vi "Get Calibration Point Auto.vi"(0 "Manipulator Interface":T3, 1 "Diagonal factor":dbl min=0.0 max=1.0, 2 "Focus and Tracking":T1, 5 "error in":errorcluster, 7 "System of Reference Interface":T2, 12 "Dialog Indicator":refnum<vi>, 13 "Calibrate button":refnum<vi>) -> (14 "Distance [um]":dbl format="%.2f", 15 "Initial [pix]":cluster{"X":sgl, "Y":sgl}, 16 "Final [pix]":cluster{"X":sgl, "Y":sgl}, 17 "Initial Reference Point [um]":cluster{"X":dbl, "Y":dbl}, 18 "Final Reference Point [um]":cluster{"X":dbl, "Y":dbl}, 19 "error out":errorcluster)   [LabVIEW 2012, in "Targeting Unit.lvlib"]
uses:
  Targeting Unit.lvlib
  <vilib>/Analysis/Matrix/Datatypes/RealMatrix.ctl
  <vilib>/Analysis/Matrix/NI_Matrix.lvlib
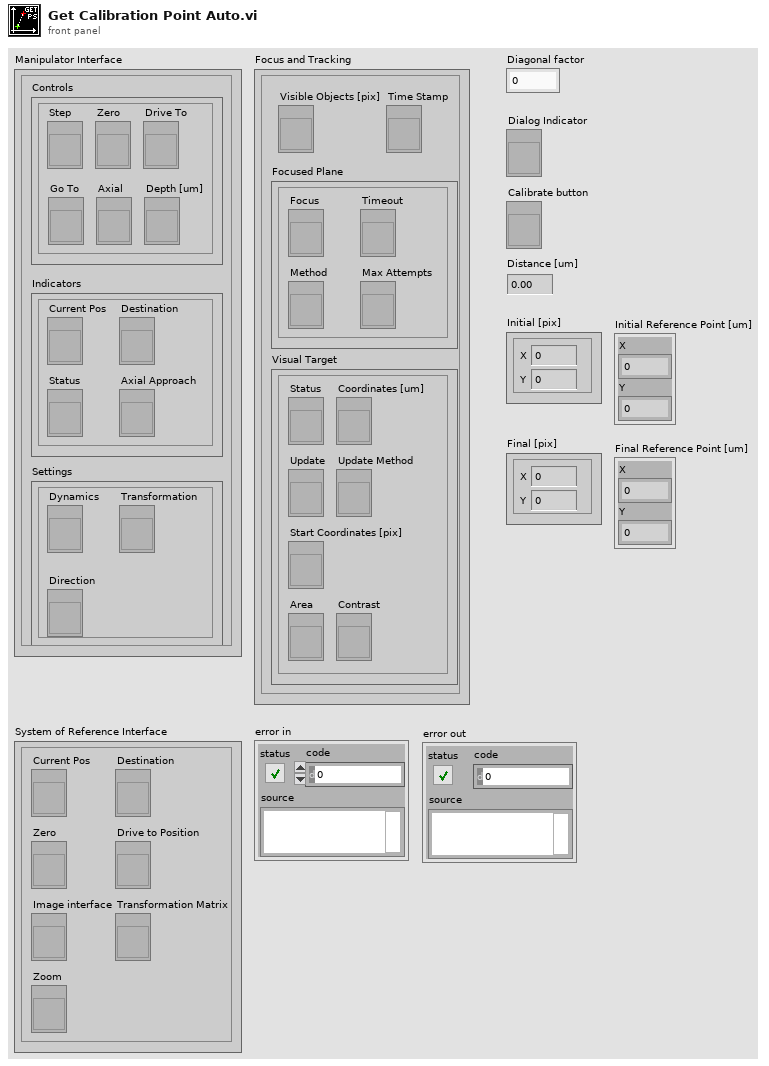
[diagram p1: front panel]
types:
  T1 = cluster{"Focused Plane":cluster{"Focus":refnum<vi>, "Timeout":refnum<vi>, "Max Attempts":refnum<vi>, "Method":refnum<vi>}, "Time Stamp":refnum<vi>, "Visual Target":cluster{"Coordinates [um]":refnum<vi>, "Status":refnum<vi>, "Update":refnum<vi>, "Update Method":refnum<vi>, "Start Coordinates [pix]":refnum<vi>, "Area":refnum<vi>, "Contrast":refnum<vi>}, "Visible Objects [pix]":refnum<vi>}
  T2 = cluster{"Current Pos":refnum<vi>, "Image interface":refnum<vi>, "Transformation Matrix":refnum<vi>, "Zero":refnum<vi>, "Destination":refnum<vi>, "Drive to Position":refnum<vi>, "Zoom":refnum<vi>}
  T3 = cluster{"Indicators":cluster{"Current Pos":refnum<vi>, "Destination":refnum<vi>, "Status":refnum<vi>, "Axial Approach":refnum<vi>}, "Settings":cluster{"Dynamics":refnum<vi>, "Transformation":refnum<vi>, "Direction":refnum<vi>}, "Controls":cluster{"Zero":refnum<vi>, "Step":refnum<vi>, "Drive To":refnum<vi>, "Go To":refnum<vi>, "Axial":refnum<vi>, "Depth [um]":refnum<vi>}}
  T4 = cluster{"X [um]":dbl, "Y [um]":dbl, "Z [um]":dbl}
  T5 = typedef "NI_Matrix.lvlib/RealMatrix.ctl" = dbl[][]
  T6 = cluster{"Area":dbl, "Centre of Mass":cluster{"X":dbl, "Y":dbl}, "Global Rectangle":cluster{"Left":dbl, "Top":dbl, "Right":dbl, "Bottom":dbl}, "Contrast":dbl}[]
  T7 = cluster{"Area":dbl, "Centre of Mass":cluster{"X":dbl, "Y":dbl}, "Global Rectangle":cluster{"Left":dbl, "Top":dbl, "Right":dbl, "Bottom":dbl}, "Contrast":dbl}
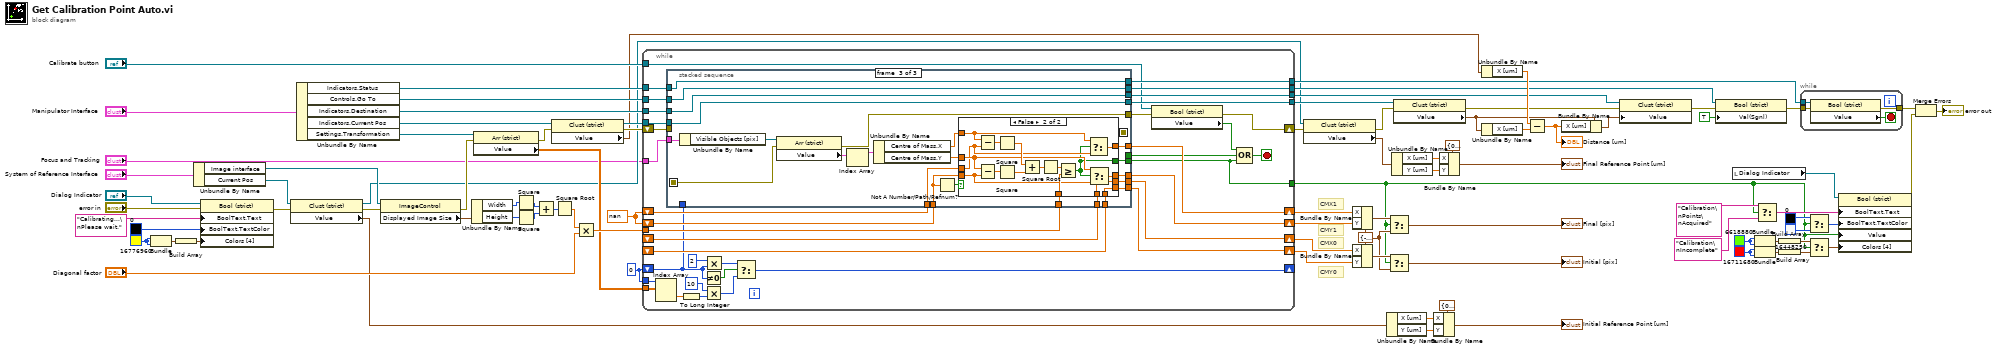
[diagram p0: block diagram]
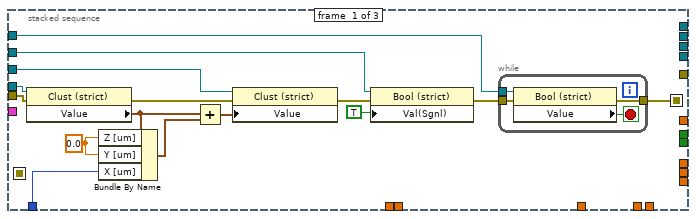
[diagram p2: hidden frame]
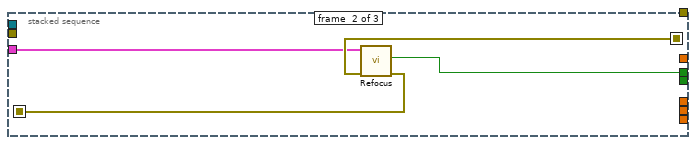
[diagram p3: hidden frame]
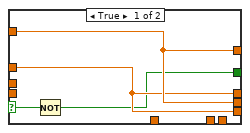
[diagram p4: hidden frame]
diagram:
  w31 = u32 16711680
  w28 = u32 6618880
  w41 = u32 16776960
  w13 = cluster{"X":i32, "Y":i32} {"X"=-1, "Y"=-1} ("Final [pix]")
  w86 = nan ("Numeric")
  w54 = 0 ("index (row)")
  # "CMY0"
  # "CMX0"
  # "CMY1"
  # "CMX1"
  n1 = Bundle(w41, w41) -> (w42:cluster{u32, u32})  [unwired: 1 in]
  n2 = Build Array(w42) -> (w38:cluster{u32, u32}[])
  n3 = Unbundle By Name("System of Reference Interface") -> ("Image interface"=w53:refnum<vi>, "Current Pos"=w46:refnum<vi>)
  n4 = property class="Bool (strict)"(reference="Dialog Indicator", error in="error in", "BoolText.Text"="Calibrating...\nPlease wait." ("Boolean Text.Text"), "BoolText.TextColor"=u32 0, "Colors [4]"=w38) -> (error out=w36:errorcluster)  [unwired: 1 out]
  n5 = property class="Clust (strict)"(reference=w46, error in=w36) -> (reference out=w43:refnum<vi>, error out=w47:errorcluster, "Value"=w11:T4)
  n6 = Unbundle By Name("Manipulator Interface") -> ("Indicators.Status"=w62:refnum<vi>, "Controls.Go To"=w63:refnum<vi>, "Indicators.Destination"=w67:refnum<vi>, "Indicators.Current Pos"=w76:refnum<vi>, "Settings.Transformation"=w74:refnum<vi>)
  n7 = property class="ImageControl"(reference=w53, error in=w47) -> (error out=w52:errorcluster, "Displayed Image Size"=w51:cluster{"Width":u32, "Height":u32})  [unwired: 1 out]
  n8 = Unbundle By Name(w51) -> ("Width"=w83:u32, "Height"=w82:u32)
  n9 = property class="Arr (strict)"(reference=w74, error in=w52) -> (error out=w55:errorcluster, "Value"=w73:T5)  [unwired: 1 out]
  n10 = Square(x=w83) -> (x^2=w89:u32)
  n11 = Square(x=w82) -> (x^2=w88:u32)
  n12 = Add(x=w89, y=w88) -> (x+y=w90:u32)
  n13 = property class="Clust (strict)"(reference=w76, error in=w55) -> (reference out=w72:refnum<vi>, error out=w75:errorcluster, "Value"=w56:T4)
  n14 = Square Root(x=w90) -> (sqrt(x)=w49:dbl)
  n15 = Multiply(x=w49, y="Diagonal factor") -> (x*y=w87:dbl)
  n16 = while {
    shift-right: [w116] -> _
    shift-left: w54 -> [w115]
    shift-right: [w110] -> w45
    shift-left: w75 -> [w118]
    shift-right: [w124] -> w81
    shift-left: w86 -> [w119]
    shift-right: [w125] -> w80
    shift-left: w86 -> [w120]
    tunnel: w87 -> [w121]
    shift-right: [w126] -> w79
    shift-left: _ -> [w122]
    shift-right: [w127] -> w78
    shift-left: _ -> [w123]
    tunnel: "Focus and Tracking" -> [w112]
    tunnel: w73 -> [w105]
    tunnel: w72 -> [w104]
    tunnel: w63 -> [w103]
    tunnel: w62 -> [w102]
    tunnel: w67 -> [w101]
    tunnel: [w100] -> w61
    tunnel: [w99] -> w60
    tunnel: [w98] -> w59
    tunnel: [w97] -> w58
    tunnel: "Calibrate button" -> [w96]
    tunnel: w54 -> [w95]
    tunnel: [w91] -> w12
    stop <- w93 stop-if-true
    n17 = Index Array(array=w105, index (row)=w95, index (col)=w95) -> (element=w108:dbl)
    n18 = stacked-sequence {
      seq-local: [w132 _ _] -> [_ w150 _]
      seq-local: [_ w149 _] -> [_ _ w161]
      tunnel: w118 -> [w141 _ _]
      tunnel: w115 -> [w142 _ _]
      tunnel: w112 -> [_ w148 w152]
      tunnel: w104 -> [w140 _ w156]
      tunnel: w103 -> [w135 _ w154]
      tunnel: w102 -> [w131 _ w153]
      tunnel: w101 -> [w130 _ w155]
      tunnel: [_ _ w172] -> w91
      tunnel: [_ _ w171] -> w127
      tunnel: [_ _ w170] -> w126
      tunnel: [_ _ w169] -> w125
      tunnel: [_ _ w168] -> w124
      tunnel: [_ _ w162] -> w111
      tunnel: w123 -> [_ _ w167]
      tunnel: w122 -> [_ _ w166]
      tunnel: w121 -> [_ _ w165]
      tunnel: w120 -> [_ _ w164]
      tunnel: w119 -> [_ _ w163]
      tunnel: [_ _ w156] -> w100
      tunnel: [_ _ w155] -> w99
      tunnel: [_ _ w154] -> w98
      tunnel: [_ _ w153] -> w97
      tunnel: [_ w147 _] -> w92
      frame #0 {
        w128 = 0.0 ("Z [um]")
        n19 = property class="Clust (strict)"(reference=w140, error in=w141) -> (error out=w139:errorcluster, "Value"=w129:T4)  [unwired: 1 out]
        n20 = Bundle By Name(cluster=w129, "Z [um]"=w128, "Y [um]"=w128, "X [um]"=w142) -> (w137:T4)
        n21 = Add(x=w129, y=w137) -> (x+y=w138:T4)
        n22 = property class="Clust (strict)"(reference=w130, error in=w139, "Value"=w138) -> (error out=w136:errorcluster)  [unwired: 1 out]
        n23 = property class="Bool (strict)"(reference=w135, error in=w136, "Val(Sgnl)"=TRUE ("Value")) -> (error out=w133:errorcluster)  [unwired: 1 out]
        n24 = while {
          tunnel: w133 -> [w146]
          tunnel: [w145] -> w132
          tunnel: w131 -> [w143]
          stop <- w144 stop-if-true
          n25 = property class="Bool (strict)"(reference=w143, error in=w146) -> (error out=w145:errorcluster, "Value"=w144:bool)  [unwired: 1 out]
        }
      }
      frame #1 {
        n26 = call "Refocus.vi"("Error In"=w150, "Focus and Tracking"=w148) -> ("Error Out"=w149:errorcluster, "Error"=w147:bool)  [unwired: 8 in]
      }
      frame #2 {
        n27 = Unbundle By Name(w152) -> ("Visible Objects [pix]"=w151:refnum<vi>)
        n28 = property class="Arr (strict)"(reference=w151, error in=w161) -> (error out=w162:errorcluster, "Value"=w157:T6)  [unwired: 1 out]
        n29 = Index Array(array=w157) -> (element=w160:T7)  [unwired: 1 in]
        n30 = Unbundle By Name(w160) -> ("Centre of Mass.X"=w158:dbl, "Centre of Mass.Y"=w159:dbl)
        n31 = Not A Number/Path/Refnum?(number/path/refnum=w164) -> (NaN/Path/Refnum?=w173:bool)
        n32 = case shown="False" w173 {
          selector: w173 -> [w175 _]
          tunnel: w159 -> [w176 w188]
          tunnel: w165 -> [_ w186]
          tunnel: w163 -> [_ w185]
          tunnel: w164 -> [_ w184]
          tunnel: w158 -> [w177 w183]
          tunnel: [w177 w182] -> w168
          tunnel: [w176 w181] -> w169
          tunnel: [w174 w178] -> w172
          tunnel: [w177 w180] -> w170
          tunnel: [w176 w179] -> w171
          tunnel: w166 -> [_ w180]
          tunnel: w167 -> [_ w179]
          frame True {
            n33 = Not(x=w175) -> (.not. x?=w174:bool)
          }
          frame False {
            n34 = Subtract(x=w183, y=w185) -> (x-y=w193:dbl)
            n35 = Subtract(x=w188, y=w184) -> (x-y=w192:dbl)
            n36 = Square(x=w193) -> (x^2=w190:dbl)
            n37 = Square(x=w192) -> (x^2=w189:dbl)
            n38 = Add(x=w190, y=w189) -> (x+y=w191:dbl)
            n39 = Square Root(x=w191) -> (sqrt(x)=w187:dbl)
            n40 = Greater Or Equal?(x=w187, y=w186) -> (x >= y?=w178:bool)
            n41 = Select(t=w183, s=w178, f=w185) -> (s? t:f=w182:dbl)
            n42 = Select(t=w188, s=w178, f=w184) -> (s? t:f=w181:dbl)
          }
        }
      }
    }
    n43 = To Long Integer(number=w108) -> (32bit integer=w107:i32)
    n44 = Not Equal To 0?(x=w115) -> (x != 0?=w117:bool)
    n45 = Multiply(x=10 ("y"), y=w107) -> (x*y=w109:i32)
    n46 = Multiply(x=2 ("y"), y=w115) -> (x*y=w113:i32)
    n47 = Select(t=w113, s=w117, f=w109) -> (s? t:f=w116:i32)
    n48 = property class="Bool (strict)"(reference=w96, error in=w111) -> (error out=w110:errorcluster, "Value"=w94:bool)  [unwired: 1 out]
    n49 = Compound Arithmetic op=OR(w94, w92, w91) -> (w93:bool)
  }
  n50 = property class="Clust (strict)"(reference=w43, error in=w45) -> (error out=w44:errorcluster, "Value"=w2:T4)  [unwired: 1 out]
  n51 = Bundle By Name(cluster=w13, "X"=w81, "Y"=w80) -> (w17:cluster{"X":i32, "Y":i32})
  n52 = Bundle By Name(cluster=w13, "X"=w79, "Y"=w78) -> (w15:cluster{"X":i32, "Y":i32})
  n53 = Unbundle By Name(w11) -> ("X [um]"=w9:dbl, "Y [um]"=w8:dbl)
  n54 = Select(t=w17, s=w12, f=w13) -> (s? t:f=→"Final [pix]":cluster{"X":i32, "Y":i32})
  n55 = Select(t=w15, s=w12, f=w13) -> (s? t:f=→"Initial [pix]":cluster{"X":i32, "Y":i32})
  n56 = Unbundle By Name(w2) -> ("X [um]"=w4:dbl, "Y [um]"=w5:dbl)
  n57 = property class="Clust (strict)"(reference=w61, error in=w44) -> (error out=w70:errorcluster, "Value"=w68:T4)  [unwired: 1 out]
  n58 = Bundle By Name(cluster=cluster{"X":dbl, "Y":dbl} {"X"=0.0, "Y"=0.0} ("Initial Reference Point [um] 2"), "X"=w9, "Y"=w8) -> (→"Initial Reference Point [um]":cluster{"X":dbl, "Y":dbl})
  n59 = Bundle By Name(cluster=cluster{"X":dbl, "Y":dbl} {"X"=0.0, "Y"=0.0} ("Initial Reference Point [um] 2"), "X"=w4, "Y"=w5) -> (→"Final Reference Point [um]":cluster{"X":dbl, "Y":dbl})
  n60 = Unbundle By Name(w56) -> ("X [um]"=w84:dbl)
  n61 = Unbundle By Name(w68) -> ("X [um]"=w85:dbl)
  n62 = Subtract(x=w84, y=w85) -> (x-y=w71:dbl)
  "Distance [um]" <- w71
  n63 = Bundle By Name(cluster=w68, "X [um]"=w71) -> (w69:T4)
  n64 = property class="Clust (strict)"(reference=w60, error in=w70, "Value"=w69) -> (error out=w64:errorcluster)  [unwired: 1 out]
  n65 = property class="Bool (strict)"(reference=w59, error in=w64, "Val(Sgnl)"=TRUE ("Value")) -> (error out=w66:errorcluster)  [unwired: 1 out]
  n66 = local read "Dialog Indicator"() -> (w18:refnum<vi>)
  n67 = Bundle(w28, w28) -> (w29:cluster{u32, u32})  [unwired: 1 in]
  n68 = Bundle(w31, w31) -> (w32:cluster{u32, u32})  [unwired: 1 in]
  n69 = Select(t="Calibration\nPoints\nAcquired" ("Boolean Text.Text"), s=w12, f="Calibration\nIncomplete" ("Boolean Text.Text")) -> (s? t:f=w24:string)
  n70 = Build Array(w29) -> (w30:cluster{u32, u32}[])
  n71 = Build Array(w32) -> (w33:cluster{u32, u32}[])
  n72 = while {
    tunnel: w66 -> [w197]
    tunnel: [w196] -> w21
    tunnel: w58 -> [w194]
    stop <- w195 stop-if-true
    n73 = property class="Bool (strict)"(reference=w194, error in=w197) -> (error out=w196:errorcluster, "Value"=w195:bool)  [unwired: 1 out]
  }
  n74 = Select(t=u32 0, s=w12, f=u32 16448250) -> (s? t:f=w27:u32)
  n75 = Select(t=w30, s=w12, f=w33) -> (s? t:f=w34:cluster{u32, u32}[])
  n76 = property class="Bool (strict)"(reference=w18, "BoolText.Text"=w24, "BoolText.TextColor"=w27, "Value"=w12, "Colors [4]"=w34) -> (error out=w19:errorcluster)  [unwired: 1 in, 1 out]
  n77 = Merge Errors(w21, w19) -> (→"error out":errorcluster)
